vi "Keithley 6517A Zero Check.vi"(1 "Zero Check":bool=TRUE, 2 "error in":T1, 3 "GPIB address":string="27") -> (0 "error out":T1)   [LabVIEW 2024]
doc: "This VI for the Keithley 6517A Electrometer allows the operator to turn the 'Zero Check' function on or off.\n\n1 or True: Zero Check On\n0 or False: Zero Check Off"
panel:
  # "ON\nOFF"
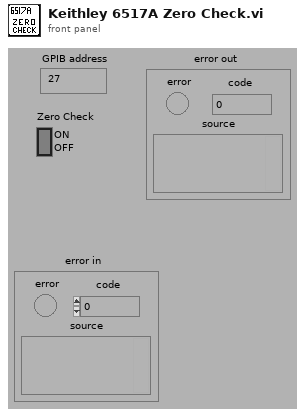
[diagram p1: front panel]
types:
  T1 = cluster{"error":bool, "code":i32, "source":string}
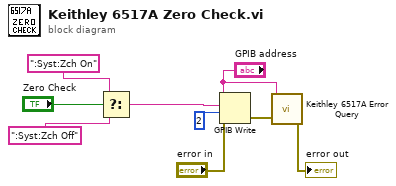
[diagram p0: block diagram]
diagram:
  n1 = Select(t=":Syst:Zch On", s="Zero Check", f=":Syst:Zch Off") -> (s? t:f=w6:string)
  n2 = GPIB Write(0:"GPIB address", 1:w6, 2:2, 3:"error in") -> (6:w1:errorcluster)  [unwired: 1 in, 1 out]
  n3 = call "Keithley 6517A Error Query.vi"("GPIB address"="GPIB address", "error in"=w1) -> ("error out"=→"error out":T1)  [unwired: 1 in, 2 out]
